vi "Create Transfer Channels.vi"(7 "GUID (Default Channel)":string="03D3BB99-1485-13A6-561D1F898F032919", 8 "error in (no error)":errorcluster, 9 "direction":T6, 10 "channels":T1[](array[typedef]) {"core"."string offset" format="%d bytes"}, 11 "Item Ref in":T5 format="%.0x") -> (0 "error out":errorcluster, 3 "Item Ref out":T5 format="%.0x", 5 "channel count":i32)   [LabVIEW 2020, in "DSF System Explorer.lvlib"]
uses:
  DSF System Explorer.lvlib
  <vilib>/NI VeriStand/Custom Device API/Custom Device Item Ref.ctl
  DSF Core.lvlibp/Typedefs/DSF Direction.ctl
  DSF Core.lvlibp/Typedefs/DSF Engine Channel Configuration.ctl
  DSF Core.lvlibp/Typedefs/Core Channel Configuration.ctl
  DSF Core.lvlibp/Typedefs/DSF Data Type.ctl
  DSF Core.lvlibp/Typedefs/DSF Settings Info.ctl
  <vilib>/NI VeriStand/Custom Device API/Custom Device Channel Type.ctl
  <vilib>/NI VeriStand/Custom Device API/Custom Device Channel.ctl
  <vilib>/NI VeriStand/Custom Device API/Custom Device API.lvlib
  Source/DSF Core.lvlibp
  DSF Core.lvlibp/Classes/Configuration/Core/Channel/Channel Configuration.lvclass
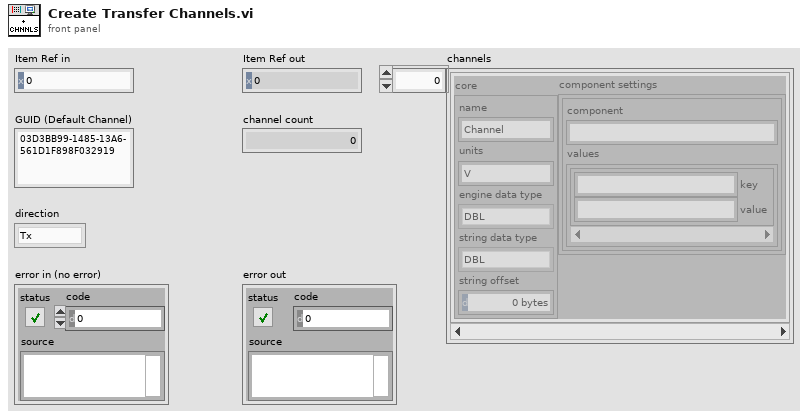
[diagram p1: front panel]
types:
  T1 = typedef "DSF Core.lvlibp/DSF Engine Channel Configuration.ctl" = cluster{"core":T2, "component settings":T4[]}
  T2 = typedef "DSF Core.lvlibp/Channel Configuration.lvclass/Core Channel Configuration.ctl" = cluster{"name":string, "units":string, "engine data type":T3, "string data type":T3, "string offset":u64}
  T3 = typedef "DSF Core.lvlibp/DSF Data Type.ctl" = enum8{"Bool", "SGL", "DBL", "I8", "I16", "I32", "I64", "U8", "U16", "U32", "U64"}
  T4 = typedef "DSF Core.lvlibp/DSF Settings Info.ctl" = cluster{"component":string, "values":cluster{"key":string, "value":string}[]}
  T5 = typedef "Custom Device API.lvlib/Custom Device Item Ref.ctl" = u64
  T6 = typedef "DSF Core.lvlibp/DSF Direction.ctl" = enum8{"Tx", "Rx"}
  T7 = typedef "Custom Device API.lvlib/Custom Device Channel Type.ctl" = enum16{"Input", "Output"}
  T8 = typedef "Custom Device API.lvlib/Custom Device Channel.ctl" = cluster{"Type":T7, "Units":string, "Default Value":dbl, "Faultable":bool, "Scalable":bool}
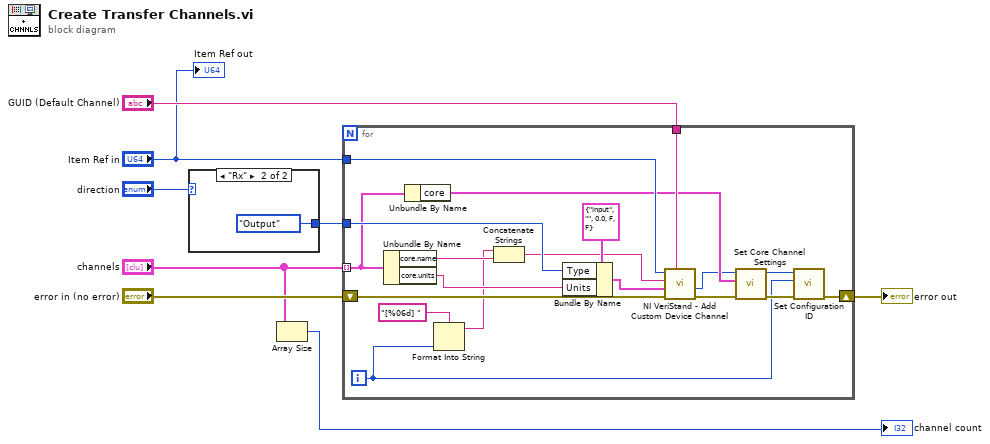
[diagram p0: block diagram]
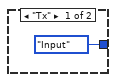
[diagram p2: hidden frame]
diagram:
  n1 = case shown="\"Rx\"" "direction" {
    tunnel: [Custom_Device_Channel_Type."Input" ("Type") Custom_Device_Channel_Type."Output" ("Type")] -> w7
    frame "Tx" {
    }
    frame "Rx" {
    }
  }
  n2 = Array Size(array="channels") -> (size(s)=→"channel count":i32)
  n3 = for {
    tunnel: "Item Ref in" -> [w23]
    tunnel: w7 -> [w27]
    tunnel: "channels" -> [w14] mode=indexing
    tunnel: "GUID (Default Channel)" -> [w26]
    shift-right: [w18] -> w6
    shift-left: "error in (no error)" -> [w20]
    i -> [w15]
    n4 = Unbundle By Name(w14) -> ("core.name"=w22:string, "core.units"=w21:string)
    n5 = Unbundle By Name(w14) -> ("core"=w13:T2)
    n6 = Format Into String(format string="[%06d] ", w15) -> (resulting string=w19:string)  [unwired: 2 in, 1 out]
    n7 = Concatenate Strings(w19, w22) -> (w25:string)
    n8 = Bundle By Name(cluster=T8 {"Type"=enum."Input", "Units"="", "Default Value"=0.0, "Faultable"=FALSE, "Scalable"=FALSE} ("Channel"), "Type"=w27, "Units"=w21) -> (w28:T8)
    n9 = call <vilib>:"NI VeriStand - Add Custom Device Channel.vi"("GUID (Default Channel)"=w26, "error in (no error)"=w20, "Channel"=w28, "Channel Name"=w25, "Parent Ref in"=w23) -> ("error out"=w17:errorcluster, "Channel Ref"=w12:T5)  [unwired: 3 in, 2 out]
    n10 = call "Set Core Channel Settings.vi"("error in (no error)"=w17, "channel configuration"=w13, "Item Ref in"=w12) -> ("error out"=w16:errorcluster, "Item Ref out"=w11:T5)  [unwired: 7 in]
    n11 = call "Set Configuration ID.vi"("error in (no error)"=w16, "Configuration ID"=w15, "Item Ref in"=w11) -> ("error out"=w18:errorcluster)  [unwired: 7 in, 1 out]
  }
  "error out" <- w6
  "Item Ref out" <- "Item Ref in"
